vi "mqttCmdCreate.vi"(8 "error in (no error)":errorcluster, 10 "messageID":u16) -> (0 "error out":errorcluster, 3 "mqttCmdPublishAck out":refnum<class "mqttCmdPublishAck.lvclass">)   [LabVIEW 2020, in "mqttCmdPublishAck.lvclass"]
uses:
  mqttCmdPublishAck.lvclass
  C:/Projects/Libraries/Gore SM 2020/mqtt-LabVIEW/src/class/mqtt/mqttCmd/mqttCmd.lvclass
  mqttTypedef/mqttMessageType.ctl
  mqttTypedef/mqttQOSlevel.ctl
  mqttCmd.lvclass/mqttCmd.ctl
  Properties/Write Datagram.vi
  mqttCmd.lvclass
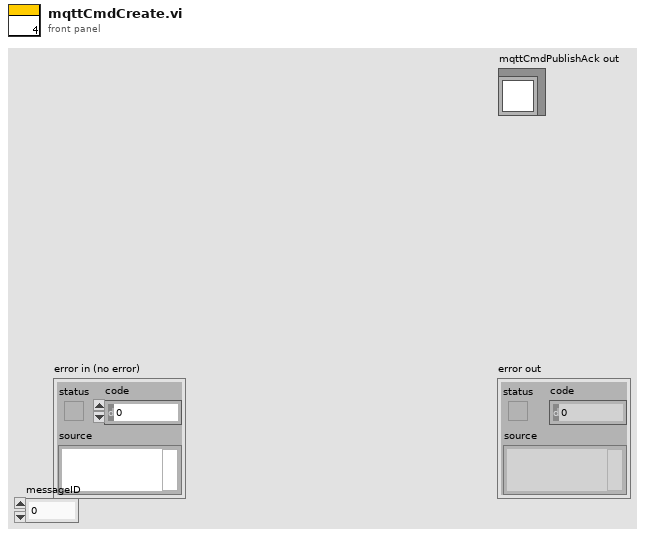
[diagram p1: front panel]
types:
  T1 = typedef "mqttQOSlevel.ctl" = enum8{"At most once", "At least once", "Exactly once", "Reserved"}
  T2 = typedef "mqttMessageType.ctl" = enum32{"Reserved", "CONNECT", "CONNACK", "PUBLISH", "PUBACK", "PUBREC", "PUBREL", "PUBCOMP", "SUBSCRIBE", "SUBACK", "UNSUBSCRIBE", "UNSUBACK", "PINGREQ", "PINGRESP", "DISCONNECT", "Reserved2"}
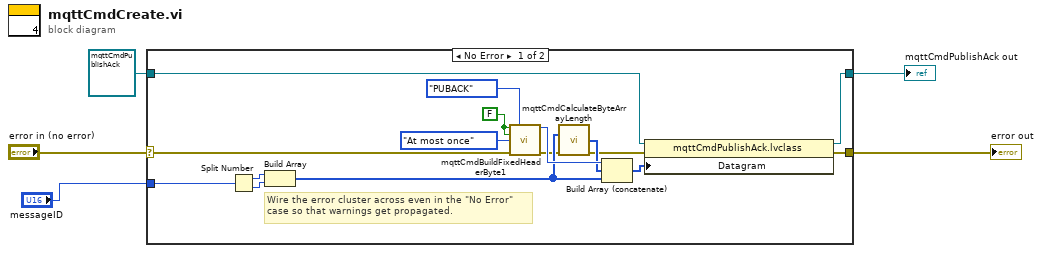
[diagram p0: block diagram]
diagram:
  n1 = case shown="No Error" "error in (no error)" {
    selector: "error in (no error)" -> [w11 w23]
    tunnel: [w7 w23] -> w4
    tunnel: [w10 w22] -> w2
    tunnel: refnum<class "mqttCmdPublishAck.lvclass"> refnum ("mqttCmdPublishAck in") -> [w21 w22]
    tunnel: "messageID" -> [w6 _]
    frame No Error {
      w12 = FALSE ("retain(F)")
      # "Wire the error cluster across even in the \"No Error\"\ncase so that warnings get propagated."
      n2 = Split Number(x=w6) -> (hi(x)=w16:u8, lo(x)=w17:u8)
      n3 = Build Array(w16, w17) -> (w15:u8[])
      n4 = call "mqttCmdBuildFixedHeaderByte1.vi"("retain(F)"=w12, "MessageType"=mqttMessageType."PUBACK", "duplicate(F)"=w12, "QoS (At most once)"=mqttQOSlevel."At most once", "error in (no error)"=w11) -> ("byte1"=w18:u8, "error out"=w14:errorcluster)  [unwired: 9 in]
      n5 = call "mqttCmdCalculateByteArrayLength.vi"("byteArry in"=w15, "error in (no error)"=w14) -> ("length out"=w13:u8[], "error out"=w8:errorcluster)  [unwired: 12 in]
      n6 = Build Array (concatenate)(w18, w13, w15) -> (w9:u8[])
      n7 = property class="mqttCmdPublishAck.lvclass"(reference=w21, error in=w8, "Datagram"=w9) -> (reference out=w10:refnum<class "mqttCmdPublishAck.lvclass">, error out=w7:errorcluster)
    }
    frame Error {
    }
  }
  "error out" <- w4
  "mqttCmdPublishAck out" <- w2
